vi "Close.vi"(8 "error in (no error)":errorcluster, 11 "Bronkhorst Settings in":T1={"VISA resource name"="", "Simulated?"=FALSE, "Smoothing Steps"=1} {"Smoothing Steps" min=1 step=1}) -> (0 "error out":errorcluster, 3 "Bronkhorst Settings out":T1={"VISA resource name"="", "Simulated?"=FALSE, "Smoothing Steps"=1} {"Smoothing Steps" min=1 step=1})   [LabVIEW 2021, in "Bronkhorst M14 Flow Meter.lvlib"]
uses:
  Bronkhorst M14 Flow Meter.lvlib
  Settings Cluster.ctl
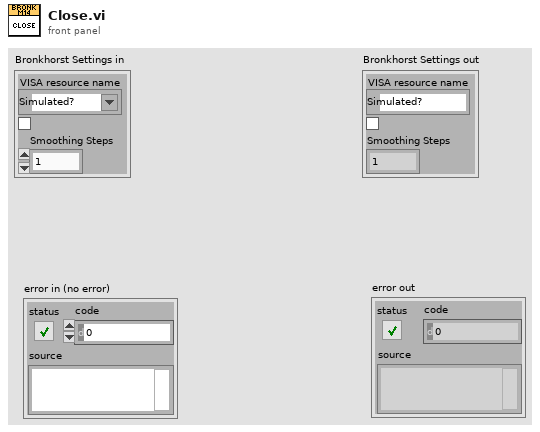
[diagram p1: front panel]
types:
  T1 = typedef "Bronkhorst M14 Flow Meter.lvlib/Settings Cluster.ctl" = cluster{"VISA resource name":refnum<visa-resource-name>, "Simulated?":bool, "Smoothing Steps":i32}
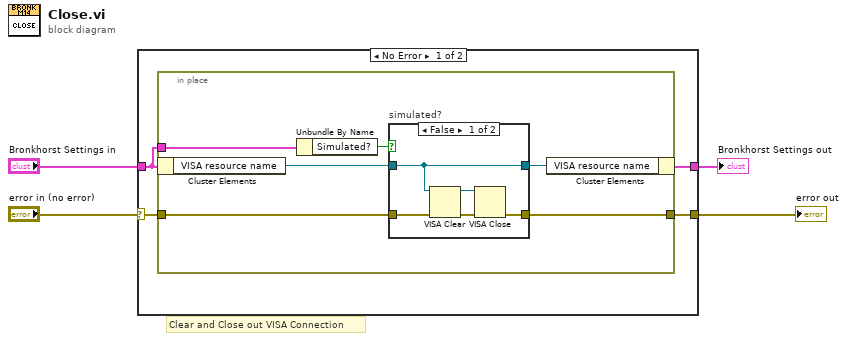
[diagram p0: block diagram]
diagram:
  # "Clear and Close out VISA Connection"
  n1 = case shown="No Error" "error in (no error)" {
    selector: "error in (no error)" -> [w8 w23]
    tunnel: [w7 w23] -> w4
    tunnel: [w5 w22] -> w1
    tunnel: "Bronkhorst Settings in" -> [w6 w22]
    frame No Error {
      n2 = in-place {
        in-place-border: w8 -> [w13]
        in-place-border: [w12] -> w7
        in-place-border: w6 -> [w11]
        n3 = in-place-cluster #1(w6) -> ("VISA resource name"=w10:refnum<visa-resource-name>)
        n4 = Unbundle By Name(w11) -> ("Simulated?"=w14:bool)
        n5 = case "simulated?" shown="False" w14 {
          tunnel: [w19 w21] -> w12
          tunnel: w13 -> [w16 w21]
          tunnel: [w18 w20] -> w9
          tunnel: w10 -> [w18 w20]
          frame False {
            n6 = VISA Clear(VISA resource name=w18, error in (no error)=w16) -> (VISA resource name out=w17:refnum<visa-resource-name>, error out=w15:errorcluster)
            n7 = VISA Close(VISA resource name=w17, error in (no error)=w15) -> (error out=w19:errorcluster)
          }
          frame True {
          }
        }
        n8 = in-place-cluster #1("VISA resource name"=w9) -> (w5:T1)
      }
    }
    frame Error {
    }
  }
  "error out" <- w4
  "Bronkhorst Settings out" <- w1
